vi "Find Baseclass.vi"(8 "Error In":errorcluster, 9 "Class.ID":i32, 10 "Table":string, 11 "connection reference":T1) -> (0 "Error Out":errorcluster, 1 "Base-Class.ID":i32, 3 "durp connection reference":T1)   [LabVIEW 2012, in "DB-Configuration.lvlib" / "ODBC-Interface.lvclass"]
doc: "Find baseclass id of items class hierarchie."
uses:
  ODBC-Interface.lvclass
  <vilib>/addons/database/Connection.llb/Conn ObjectReference.ctl
  <vilib>/addons/database/_DB Variant To Data/Database Variant To Data.xnode
  <vilib>/addons/database/NI_Database_API.lvlib
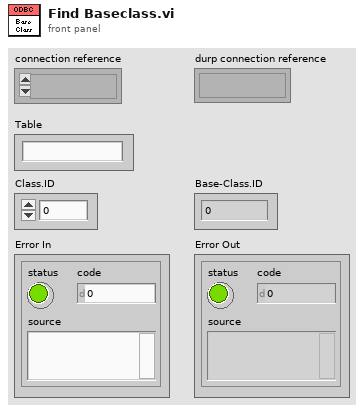
[diagram p1: front panel]
types:
  T1 = typedef "NI_Database_API.lvlib/Conn ObjectReference.ctl" = refnum<k1>
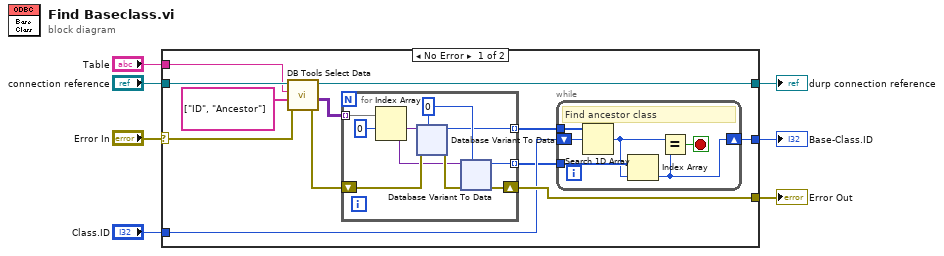
[diagram p0: block diagram]
diagram:
  n1 = case shown="No Error" "Error In" {
    selector: "Error In" -> [w8 w100]
    tunnel: "connection reference" -> [w17 w101]
    tunnel: [w16 w101] -> w6
    tunnel: [w14 w100] -> w5
    tunnel: "Table" -> [w13 _]
    tunnel: "Class.ID" -> [w12 _]
    tunnel: [w9 _] -> w3
    frame No Error {
      n2 = call <vilib>:"DB Tools Select Data.vi"("error in (no error)"=w8, "columns"=string[] ["ID", "Ancestor"], "table"=w13, "connection reference"=w17) -> ("error out"=w15:errorcluster, "data"=w18:variant[][], "connection reference out"=w16:T1)  [unwired: 2 in]
      n3 = for {
        tunnel: w18 -> [w35] mode=indexing
        tunnel: [w28] -> w11 mode=indexing
        tunnel: [w27] -> w10 mode=indexing
        shift-right: [w26] -> w14
        shift-left: w15 -> [w32]
        w29 = 0
        n4 = Index Array(array=w35, index #1=0 ("index")) -> (element #1=w33:variant, element #2=w30:variant)  [unwired: 1 in]
        n5 = xnode "Database Variant To Data"("database variant"=w33, "error in (no error)"=w32, "type"=w29) -> ("data"=w28:i32, "error out"=w31:errorcluster)
        n6 = xnode "Database Variant To Data"("database variant"=w30, "error in (no error)"=w31, "type"=w29) -> ("data"=w27:i32, "error out"=w26:errorcluster)
      }
      n7 = while {
        tunnel: w11 -> [w24]
        tunnel: w10 -> [w23]
        shift-right: [w20] -> w9
        shift-left: w12 -> [w25]
        stop <- w21 stop-if-true
        # "Find ancestor class"
        n8 = Search 1D Array(1D array=w24, element=w25) -> (index of element=w22:i32)  [unwired: 1 in]
        n9 = Index Array(array=w23, index=w22) -> (element=w20:i32)
        n10 = Equal?(x=w22, y=w20) -> (x = y?=w21:bool)
      }
    }
    frame Error {
    }
  }
  "durp connection reference" <- w6
  "Error Out" <- w5
  "Base-Class.ID" <- w3
